vi "Test TDK 20-38.vi"() -> ()   [LabVIEW 2023, in "TDK20-38 API.lvlib"]
uses:
  TDK20-38 API.lvlib
panel:
  out "error out":errorcluster
  out "Output Voltage":dbl format="%.4f"
  in  "error in":errorcluster
  in  "NI MAX name":string
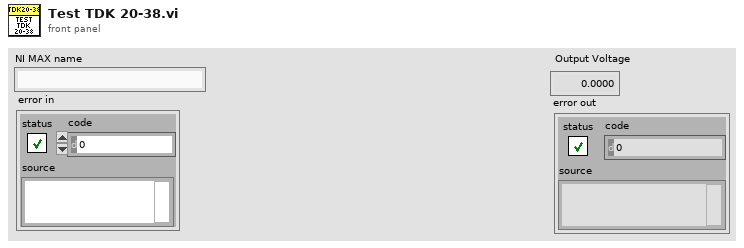
[diagram p1: front panel]
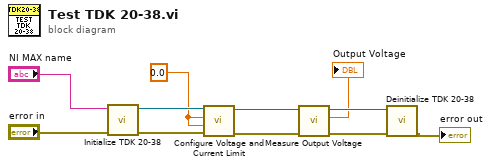
[diagram p0: block diagram]
diagram:
  w7 = 0.0 ("Voltage Limit")
  n1 = call "Initialize TDK 20-38.vi"("error in (no error)"="error in", "NI MAX name"="NI MAX name") -> ("error out"=w8:errorcluster, "VISA out"=w9:refnum<visa-resource-name>)  [unwired: 8 in]
  n2 = call "Configure Voltage and Current Limit.vi"("error"=w8, "Current Limit"=w7, "Voltage Limit"=w7, "VISA in"=w9) -> ("error out"=w5:errorcluster, "VISA out"=w6:refnum<visa-resource-name>)  [unwired: 6 in]
  n3 = call "Measure Output Voltage.vi"("error"=w5, "VISA in"=w6) -> ("error out"=w3:errorcluster, "Output Voltage"=→"Output Voltage":dbl, "VISA out"=w4:refnum<visa-resource-name>)  [unwired: 7 in]
  n4 = call "Deinitialize TDK 20-38.vi"("error"=w3, "VISA name"=w4) -> ("error out"=→"error out":errorcluster)  [unwired: 9 in]
